vi "Test Write Bit.vi"() -> ()   [LabVIEW 2014]
uses:
  ALPHA5 RS485/typedefs/Port Selection Info.ctl
  ALPHA5 RS485/ALPHA5 RS485.lvlib
panel:
  out "ON/OFF 2":bool
  in  "ON/OFF":bool
  out "error out":errorcluster
  out "CRC Match":bool
  out "FC":u8
  in  "Address":u16=65535 format="%.0x"
  in  "error in (no error)":errorcluster caption="error in（no error）"
  in  "Port Selection Info In":T1={"Port Name"="", "Amplifier Num"=1, "Baud Rate"=38400, "Char Formation"=enum."0"} {"Baud Rate" items=["38400"=38400, "19200"=19200, "9600"=9600, "115200"=0]; "Amplifier Num" max=31}
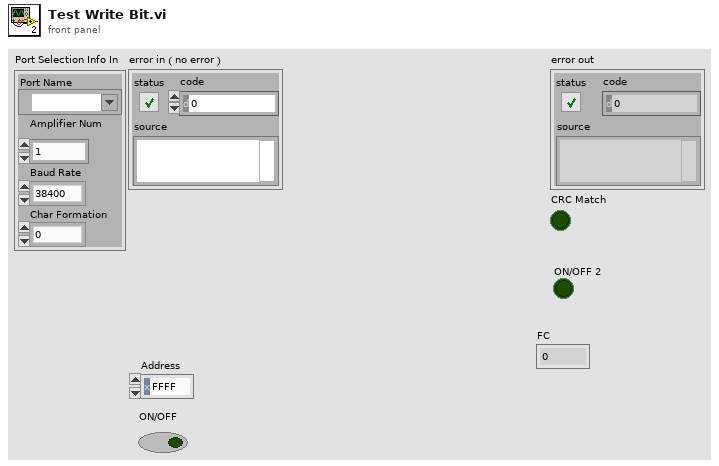
[diagram p1: front panel]
types:
  T1 = typedef "ALPHA5 RS485.lvlib/Port Selection Info.ctl" = cluster{"Port Name":refnum<visa-resource-name>, "Amplifier Num":u8, "Baud Rate":u32, "Char Formation":enum16{"0", "1", "2", "3", "4", "5"}}
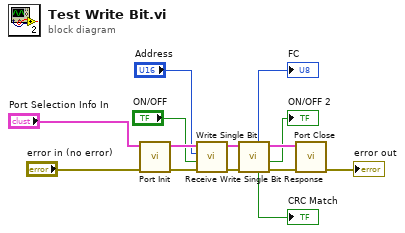
[diagram p0: block diagram]
diagram:
  n1 = call "Port Init.vi"("error in (no error)"="error in (no error)", "Port Selection Info In"="Port Selection Info In") -> ("error out"=w6:errorcluster, "Port Selection Info Out"=w7:T1)  [unwired: 8 in]
  n2 = call "Write Single Bit.vi"("error in (no error)"=w6, "ON/OFF"="ON/OFF", "Address"="Address", "Port Selection Info"=w7) -> ("error out"=w13:errorcluster, "Port Selection Info Out"=w14:T1)  [unwired: 6 in]
  n3 = call "Receive Write Single Bit Response.vi"("error in (no error)"=w13, "Port Selection Info"=w14) -> ("error out"=w9:errorcluster, "ON/OFF"=→"ON/OFF 2":bool, "Port Selection Info Out"=w10:T1, "CRC Match"=→"CRC Match":bool, "FC"=→"FC":u8)  [unwired: 3 in, 2 out]
  n4 = call "Port Close.vi"("error in (no error)"=w9, "Port Selection Info In"=w10) -> ("error out"=→"error out":errorcluster)  [unwired: 9 in]
